vi "Measure Gain and Phase.vi"(8 "error out输入":errorcluster caption="error out", 10 "Ch2":waveform(dbl) caption="waveform", 11 "Ch1":waveform(dbl) caption="waveform") -> (0 "错误输出":errorcluster, 2 "Phase":dbl, 3 "Gain (dB)":dbl)   [LabVIEW 2019]
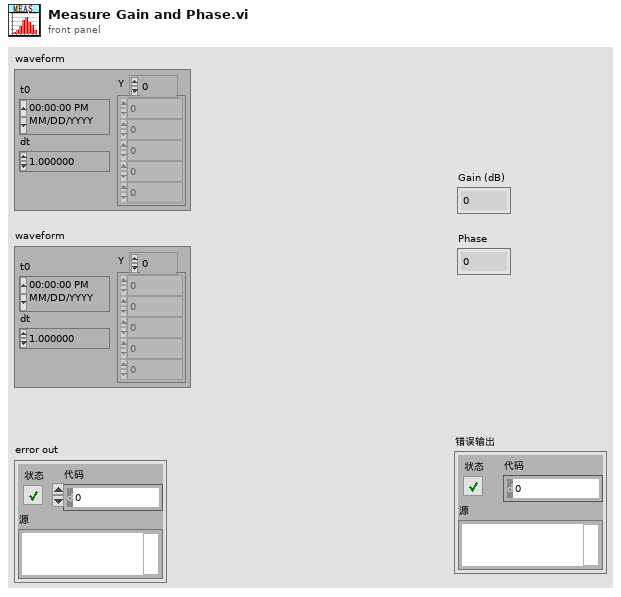
[diagram p1: front panel]
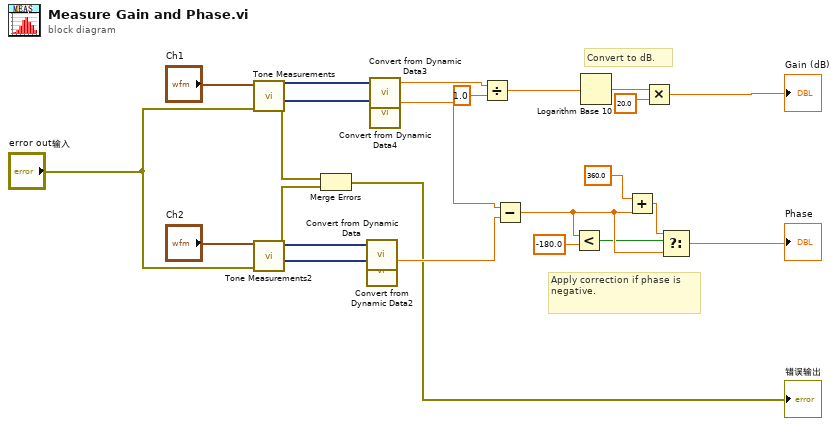
[diagram p0: block diagram]
diagram:
  # "Convert to dB."
  # "Apply correction if phase is negative."
  n1 = call "Tone Measurements"("error in (no error)"="error out输入", "Signals"="Ch1") -> ("error out"=w6:errorcluster, "Phase"=w18:dynamicdata, "Amplitude"=w17:dynamicdata)  [unwired: 7 in]
  n2 = call "Tone Measurements2"("error in (no error)"="error out输入", "Signals"="Ch2") -> ("error out"=w7:errorcluster, "Phase"=w10:dynamicdata, "Amplitude"=w9:dynamicdata)  [unwired: 7 in]
  n3 = Merge Errors(w6, w7) -> (→"错误输出":errorcluster)
  n4 = call "Convert from Dynamic Data"("Dynamic Data Type"=w9) -> ()  [unwired: 3 in, 1 out]
  n5 = call "Convert from Dynamic Data2"("Dynamic Data Type"=w10) -> ("Scalar"=w23:dbl)  [unwired: 3 in]
  n6 = call "Convert from Dynamic Data3"("Dynamic Data Type"=w17) -> ("Scalar"=w19:dbl)  [unwired: 3 in]
  n7 = call "Convert from Dynamic Data4"("Dynamic Data Type"=w18) -> ("Scalar"=w22:dbl)  [unwired: 3 in]
  n8 = Divide(x=w19, y=1.0) -> (x/y=w13:dbl)
  n9 = Subtract(x=w22, y=w23) -> (x-y=w24:dbl)
  n10 = Less?(x=w24, y=-180.0) -> (x < y?=w21:bool)
  n11 = Logarithm Base 10(1:w13) -> (0:w11:dbl)
  n12 = Add(x=360.0, y=w24) -> (x+y=w16:dbl)
  n13 = Multiply(x=w11, y=20.0 ("x")) -> (x*y=→"Gain (dB)":dbl)
  n14 = Select(t=w16, s=w21, f=w24) -> (s? t:f=→"Phase":dbl)
